vi "stuff_bytes.vi"(11 "ByteArrayIn":u8[](array[numeric])=[17, 19] format="%x") -> (3 "StuffedDataOut":u8[](array[numeric])=[17, 19] format="%x")   [LabVIEW 2019]
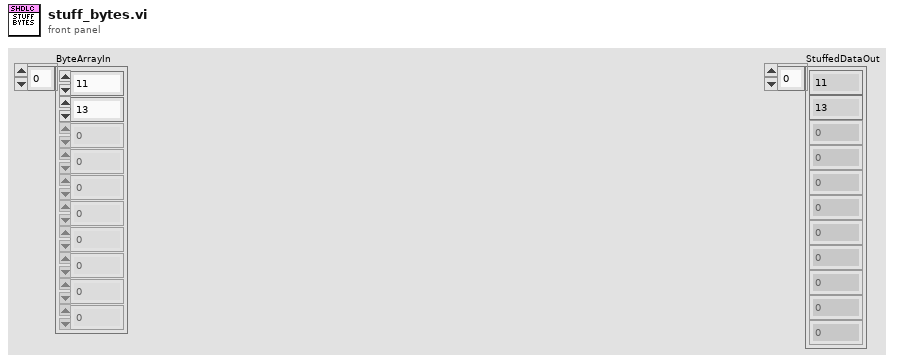
[diagram p1: front panel]
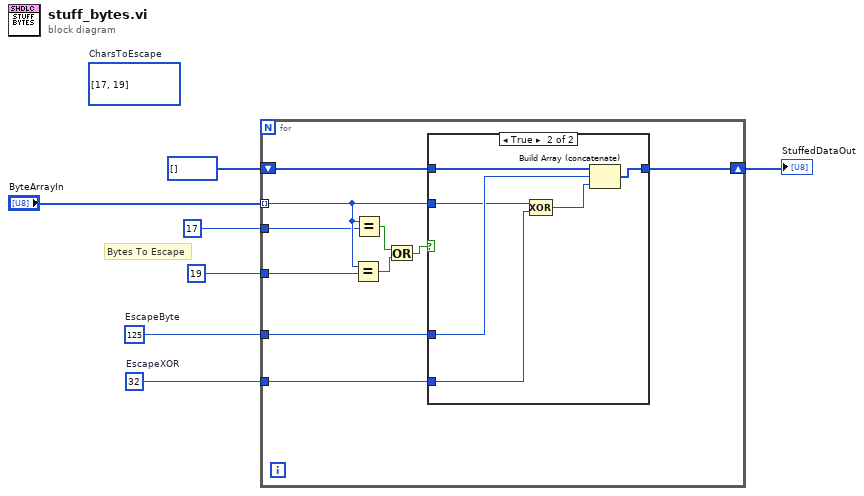
[diagram p0: block diagram]
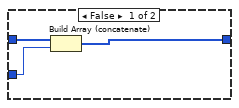
[diagram p2: hidden frame]
diagram:
  (unwired) u8[] [17, 19]  # CharsToEscape
  w4 = u8 32  # EscapeXOR
  w5 = u8 125  # EscapeByte
  # "Bytes To Escape"
  n1 = for {
    tunnel: "ByteArrayIn" -> [w16] mode=indexing
    shift-right: [w15] -> w3
    shift-left: u8[] [] ("ByteArrayIn 2") -> [w17]
    tunnel: w5 -> [w11]
    tunnel: w4 -> [w10]
    tunnel: u8 19 ("Char to Escape") -> [w9]
    tunnel: u8 17 ("Char to Escape") -> [w8]
    n2 = Equal?(x=w16, y=w9) -> (x = y?=w13:bool)
    n3 = Equal?(x=w16, y=w8) -> (x = y?=w12:bool)
    n4 = Or(x=w12, y=w13) -> (x .or. y?=w14:bool)
    n5 = case shown="True" w14 {
      tunnel: w17 -> [w20 w26]
      tunnel: w16 -> [w19 w23]
      tunnel: [w18 w21] -> w15
      tunnel: w11 -> [_ w25]
      tunnel: w10 -> [_ w24]
      frame False {
        n6 = Build Array (concatenate)(w20, w19) -> (w18:u8[])
      }
      frame True {
        n7 = Compound Arithmetic op=XOR(w23, w24) -> (w22:u8)
        n8 = Build Array (concatenate)(w26, w25, w22) -> (w21:u8[])
      }
    }
  }
  "StuffedDataOut" <- w3
